vi "meth.Constructor.vi"(11 "error in":errorcluster) -> (4 "GLue out":refnum<class "class.GLue.lvclass">, 15 "error out":errorcluster)   [LabVIEW 2014, in "GLue.lvlib" / "class.GLue.lvclass"]
uses:
  class.GLue.lvclass
  class.GLue.lvclass/class.GLue.ctl
  vi.GlueInternalModule.vi
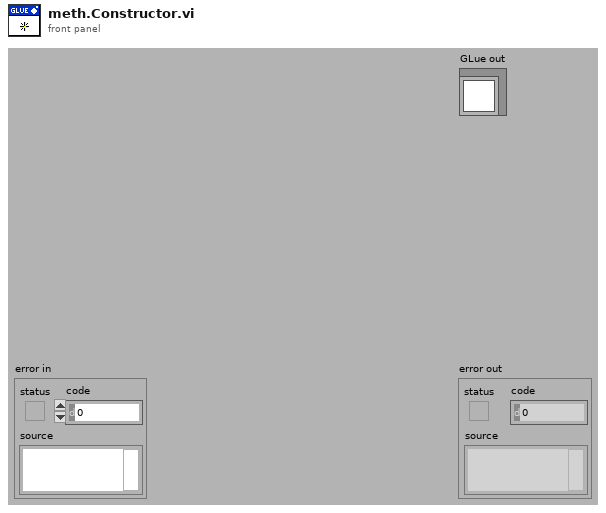
[diagram p1: front panel]
types:
  T1 = cluster{"StreamReader":refnum<vi>, "UserData":variant}
  T2 = typedef "Semaphore RefNum" = refnum<k1>
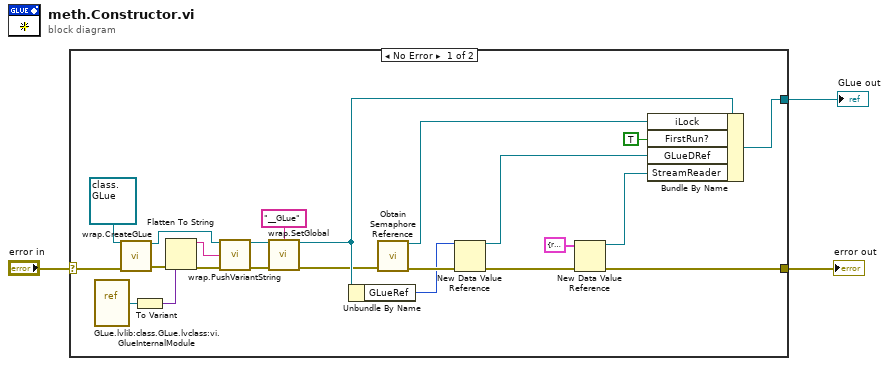
[diagram p0: block diagram]
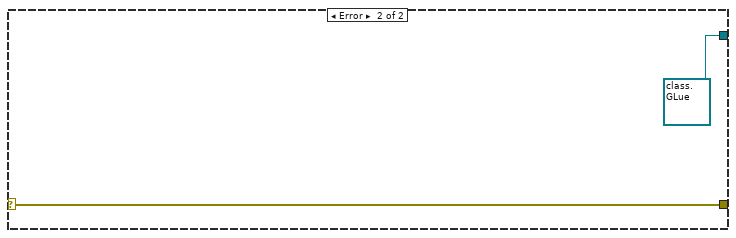
[diagram p2: hidden frame]
diagram:
  n1 = case shown="No Error" "error in" {
    selector: "error in" -> [w20 w28]
    tunnel: [w17 w28] -> w2
    tunnel: [w26 refnum<class "class.GLue.lvclass"> refnum ("class.GLue out")] -> w1
    frame No Error {
      n2 = vi-ref "GLue.lvlib:class.GLue.lvclass:vi.GlueInternalModule.vi"() -> (w5:refnum<vi>)
      n3 = call "wrap.CreateGLue.vi"("class.GLue in"=refnum<class "class.GLue.lvclass"> refnum ("GLue in"), "error in (no error)"=w20) -> ("class.GLue out"=w10:refnum<class "class.GLue.lvclass">, "error out"=w13:errorcluster)  [unwired: 12 in]
      n4 = To Variant(anything=w5) -> (Variant=w4:variant)
      n5 = Flatten To String(anything=w4, error in (no error)=w13) -> (data string=w11:string, error out=w12:errorcluster)  [unwired: 2 in, 1 out]
      n6 = call "wrap.PushVariantString.vi"("class.GLue in"=w10, "VariantString"=w11, "error in (no error)"=w12) -> ("class.GLue out"=w8:refnum<class "class.GLue.lvclass">, "error out"=w9:errorcluster)  [unwired: 11 in]
      n7 = call "wrap.SetGlobal.vi"("class.GLue in"=w8, "Name"="__GLue", "error in (no error)"=w9) -> ("class.GLue out"=w7:refnum<class "class.GLue.lvclass">, "error out"=w6:errorcluster)  [unwired: 11 in]
      n8 = Unbundle By Name(w7) -> ("GLueRef"=w22:i64)
      n9 = call <vilib>:"Obtain Semaphore Reference.vi"("error in (no error)"=w6) -> ("error out"=w23:errorcluster, "semaphore"=w25:T2)  [unwired: 4 in, 1 out]
      n10 = New Data Value Reference(data value=w22, error in=w23) -> (data value reference=w21:refnum<data-value>, error out=w18:errorcluster)
      n11 = New Data Value Reference(data value=T1 {"StreamReader"=refnum, "UserData"=variant}, error in=w18) -> (data value reference=w16:refnum<data-value>, error out=w17:errorcluster)
      n12 = Bundle By Name(cluster=w7, "iLock"=w25, "FirstRun?"=TRUE, "GLueDRef"=w21, "StreamReader"=w16) -> (w26:refnum<class "class.GLue.lvclass">)
    }
    frame Error {
    }
  }
  "error out" <- w2
  "GLue out" <- w1
